vi "benchmark sequence structure.vi"() -> ()   [LabVIEW 2013, in "NISE Tools Drop Templates.lvlib"]
uses:
  NISE Tools Drop Templates.lvlib
panel:
  out "dT":dbl
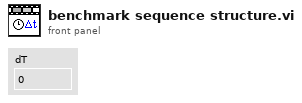
[diagram p1: front panel]
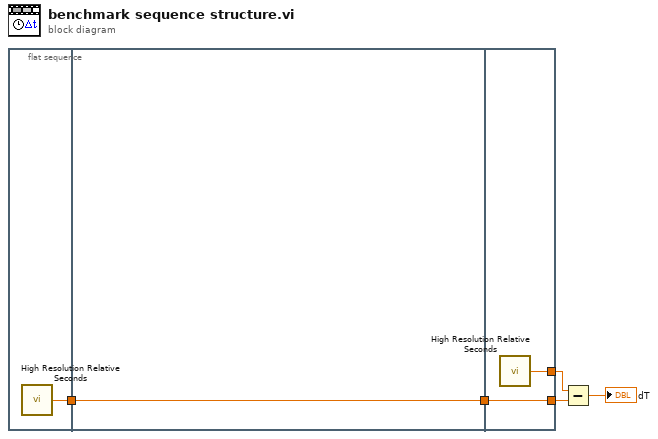
[diagram p0: block diagram]
diagram:
  n1 = flat-sequence {
    tunnel: [w6] -> w5
    tunnel: w5 -> [w7]
    tunnel: [w7] -> w4
    tunnel: [w9] -> w3
    tunnel: w4 -> [w9]
    tunnel: [w8] -> w2
    frame #0 {
      n2 = call <vilib>:"High Resolution Relative Seconds.vi"() -> ("relative seconds"=w6:dbl)
    }
    frame #1 {
    }
    frame #2 {
      n3 = call <vilib>:"High Resolution Relative Seconds.vi"() -> ("relative seconds"=w8:dbl)
    }
  }
  n4 = Subtract(x=w2, y=w3) -> (x-y=→"dT":dbl)
